vi "Stop Work.vi"(8 "error in (no error)":errorcluster, 9 "Reply":bool=TRUE, 10 "Reply to":refnum<class "Stop Response Msg.lvclass">, 11 "Measure Object in":refnum<class "Worker.lvclass">) -> (0 "error out":errorcluster, 3 "Measure Object out":refnum<class "Worker.lvclass">)   [LabVIEW 2016, in "Worker.lvclass"]
uses:
  Worker.lvclass
  C:/github/LabActor/Template Module/Template Module.lvclass
  Controllers/Process Controller Messages/Stop Response Msg/Stop Response Msg.lvclass
  Worker State.ctl
  Worker.lvclass/Worker.ctl
  Template Module/Template Module.lvclass/Template Module.ctl
  Controllers/Process Controller Messages/Stop Response Msg/Stop Response Msg.lvclass/Stop Response Msg.ctl
  Controllers/Process Controller Messages/Stop Response Msg/Write Name.vi
  Template Module/Write State.vi
  Template Module/Read Name.vi
  Write Pause requested.vi
  Write Paused.vi
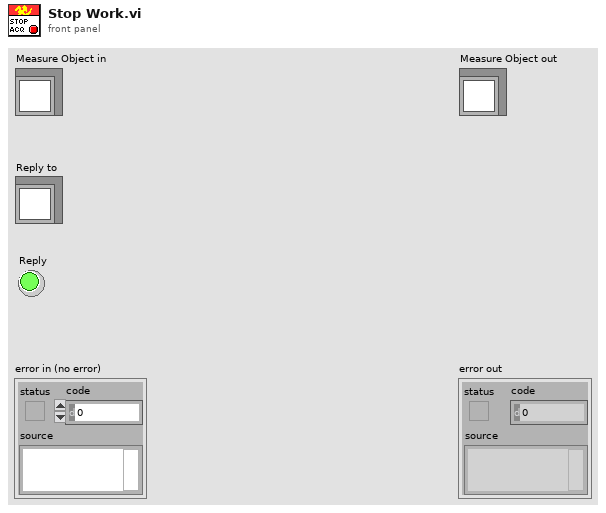
[diagram p1: front panel]
types:
  T1 = typedef "Worker State.ctl" = enum16{"Idle", "Starting", "Working", "Stopping"}
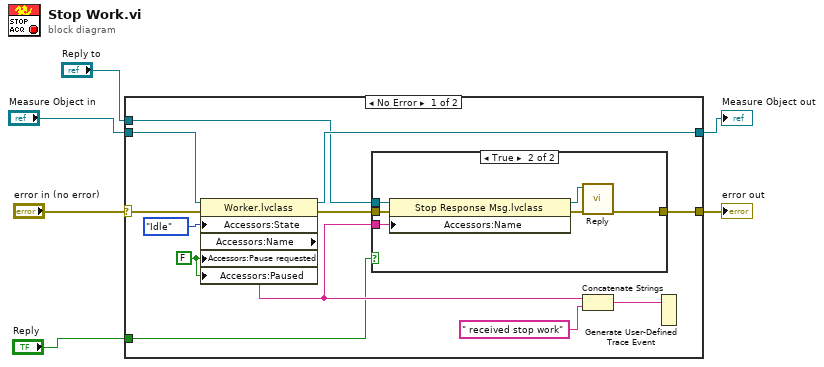
[diagram p0: block diagram]
diagram:
  n1 = case shown="No Error" "error in (no error)" {
    selector: "error in (no error)" -> [w16 w27]
    tunnel: [w9 w27] -> w5
    tunnel: [w17 w26] -> w3
    tunnel: "Measure Object in" -> [w18 w26]
    tunnel: "Reply to" -> [w12 _]
    tunnel: "Reply" -> [w8 _]
    frame No Error {
      w7 = FALSE ("Pause requested")
      n2 = property class="Worker.lvclass"(reference=w18, error in=w16, "Accessors:State"=Worker_State."Idle" ("State"), "Accessors:Pause requested"=w7, "Accessors:Paused"=w7) -> (reference out=w17:refnum<class "Worker.lvclass">, error out=w10:errorcluster, "Accessors:Name"=w11:string)
      n3 = case shown="True" w8 {
        tunnel: w12 -> [_ w25]
        tunnel: w11 -> [_ w24]
        tunnel: w10 -> [w19 w23]
        tunnel: [w19 w20] -> w9
        frame False {
        }
        frame True {
          n4 = property class="Stop Response Msg.lvclass"(reference=w25, error in=w23, "Accessors:Name"=w24) -> (reference out=w22:refnum<class "Stop Response Msg.lvclass">, error out=w21:errorcluster)
          n5 = call-dynamic "Reply.vi"("error in (no error)"=w21, "Self-addressed Msg in"=w22) -> ("error out"=w20:errorcluster)  [unwired: 8 in, 1 out]
        }
      }
      n6 = Concatenate Strings(w11, " received stop work" ("string")) -> (w14:string)
      n7 = Generate User-Defined Trace Event(2:w14) -> ()  [unwired: 1 in]
    }
    frame Error {
    }
  }
  "error out" <- w5
  "Measure Object out" <- w3
